vi "Serve Buffer to Connection.vi"(8 "error in (no error)":errorcluster, 10 "Buffer":refnum<class "Buffer.lvclass">, 11 "connection ID in":refnum<k5>) -> (0 "error out":errorcluster, 3 "connection ID out":refnum<k5>)   [LabVIEW 2017, in "DSF Core.lvlib" / "Data Server Thread.lvclass"]
uses:
  Data Server Thread.lvclass
  Buffer/Buffer.lvclass
  C:/Program Files (x86)/National Instruments/LabVIEW 2017/vi.lib/NI/Memory Manager/Classes/Pointer/Pointer.lvclass
  <vilib>/NI/Memory Manager/Classes/Pointer/Pointer.lvclass/Pointer.ctl
  <vilib>/NI/Memory Manager/Classes/Pointer/Get Address.vi
  <vilib>/NI/Memory Manager/Classes/Pointer/Pointer.lvclass
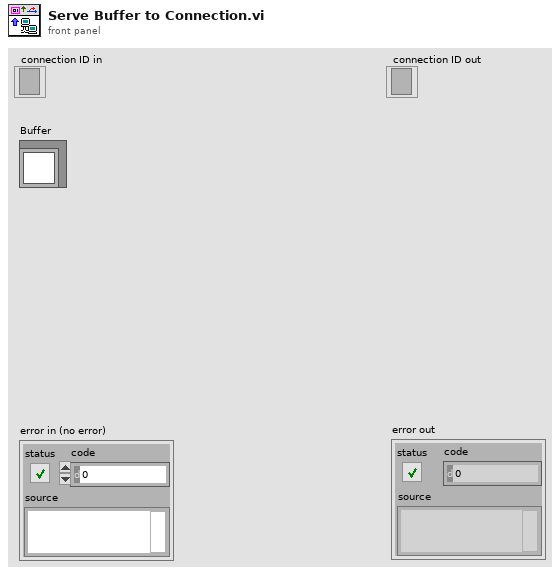
[diagram p1: front panel]
types:
  T1 = enum16{"big-endian, network order", "native, host order", "little-endian"}
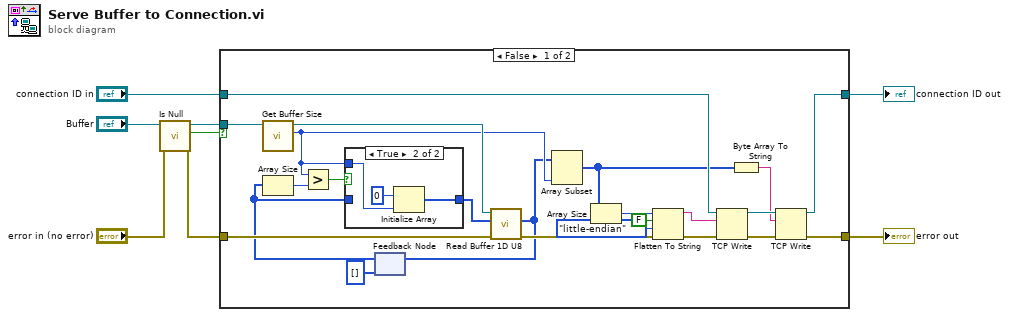
[diagram p0: block diagram]
diagram:
  n1 = call <vilib>:"Is Null.vi"("error in (no error)"="error in (no error)", "Pointer in"="Buffer") -> ("error out"=w2:errorcluster, "null?"=w1:bool, "Pointer out"=w4:refnum<class "Buffer.lvclass">)  [unwired: 7 in]
  n2 = case shown="False" w1 {
    tunnel: [w19 w36] -> w8
    tunnel: "connection ID in" -> [w28 w37]
    tunnel: [w20 w37] -> w6
    tunnel: w4 -> [w25 _]
    tunnel: w2 -> [w24 w36]
    frame False {
      n3 = call "Get Buffer Size.vi"("Buffer in"=w25) -> ("buffer size"=w17:u64, "Buffer out"=w26:refnum<class "Buffer.lvclass">)  [unwired: 9 in]
      n4 = feedback #1(u8[] []) -> (w23:u8[])
      n5 = Array Size(array=w23) -> (size(s)=w30:i32)
      n6 = Greater?(x=w17, y=w30) -> (0:w29:bool)
      n7 = case shown="True" w29 {
        tunnel: [w32 w34] -> w27
        tunnel: w23 -> [w32 _]
        tunnel: w17 -> [_ w33]
        frame False {
        }
        frame True {
          n8 = Initialize Array(u8 0, w33) -> (w34:u8[])
        }
      }
      n9 = call "Read Buffer 1D U8.vi"("error in (no error)"=w24, "dst array in"=w27, "Buffer in"=w26) -> ("error out"=w14:errorcluster, "dst array out"=w10:u8[])  [unwired: 5 in, 2 out]
      n10 = feedback-in #1(w10) -> ()
      n11 = Array Subset(array=w10, length=w17) -> (w11:u8[])  [unwired: 1 in]
      n12 = Array Size(array=w11) -> (size(s)=w15:i32)
      n13 = Flatten To String(anything=w15, prepend array or string size? (T)=FALSE, byte order (0:big-endian, network order)=T1."little-endian", error in (no error)=w14) -> (data string=w9:string, error out=w13:errorcluster)  [unwired: 1 out]
      n14 = TCP Write(connection ID=w28, data in=w9, error in (no error)=w13) -> (connection ID out=w21:refnum<k5>, error out=w22:errorcluster)  [unwired: 1 in, 1 out]
      n15 = Byte Array To String(unsigned byte array=w11) -> (string=w18:string)
      n16 = TCP Write(connection ID=w21, data in=w18, error in (no error)=w22) -> (connection ID out=w20:refnum<k5>, error out=w19:errorcluster)  [unwired: 1 in, 1 out]
    }
    frame True {
    }
  }
  "error out" <- w8
  "connection ID out" <- w6
